vi "读取-设备绑定信息.vi"(8 "error in (no error)":errorcluster caption="错误输入（无错误）", 11 "设备终端输入":refnum<class "设备终端.lvclass">) -> (0 "error out":errorcluster caption="错误输出", 2 "设备绑定信息":T1, 3 "设备终端输出":refnum<class "设备终端.lvclass">)   [LabVIEW 2013, in "设备终端.lvclass"]
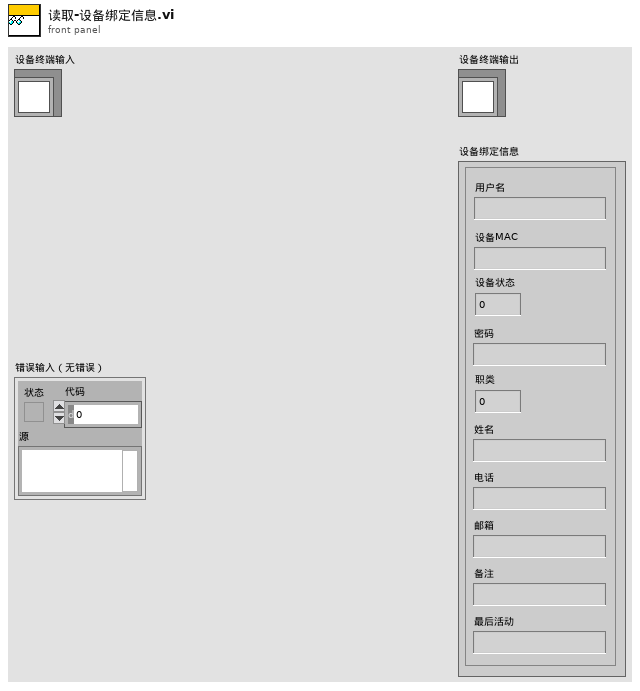
[diagram p1: front panel]
types:
  T1 = cluster{"用户名":string, "设备MAC":string, "设备状态":dbl, "密码":string, "职类":dbl, "姓名":string, "电话":string, "邮箱":string, "备注":string, "最后活动":string}
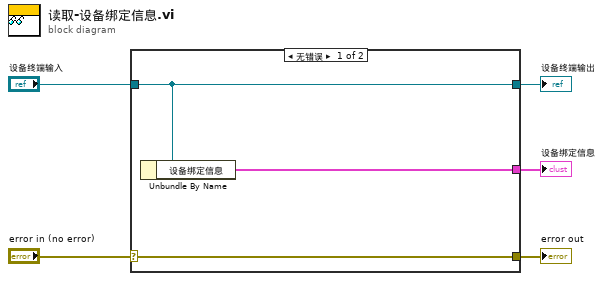
[diagram p0: block diagram]
diagram:
  n1 = case shown="无错误" "error in (no error)" {
    selector: "error in (no error)" -> [w8 w9]
    tunnel: [w8 w9] -> w4
    tunnel: [w7 w10] -> w2
    tunnel: "设备终端输入" -> [w7 w10]
    tunnel: [w6 _] -> w1
    frame No Error {
      n2 = Unbundle By Name(w7) -> ("设备绑定信息"=w6:T1)
    }
    frame Error {
    }
  }
  "error out" <- w4
  "设备终端输出" <- w2
  "设备绑定信息" <- w1
